vi "Place HDI.vi"(8 "error in (no error)":errorcluster, 9 "Slot Number":dbl, 10 "Chuck Number":dbl, 11 "PickupTool Class in":refnum<class "PickupTool Class.lvclass">) -> (0 "error out":errorcluster, 3 "PickupTool Class out":refnum<class "PickupTool Class.lvclass">)   [LabVIEW 2011, in "PickupTool Class.lvclass"]
uses:
  PickupTool Class.lvclass
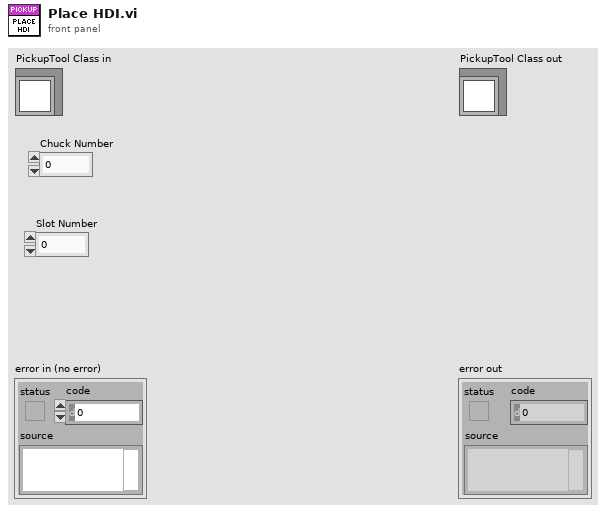
[diagram p1: front panel]
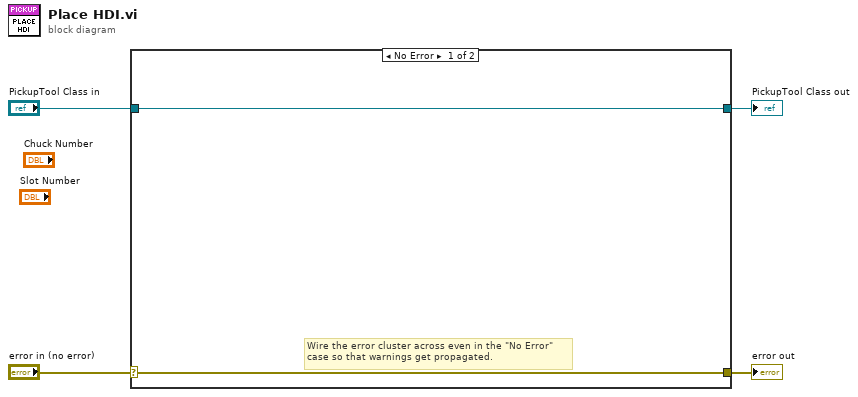
[diagram p0: block diagram]
diagram:
  n1 = case shown="No Error" "error in (no error)" {
    selector: "error in (no error)" -> [w5 w8]
    tunnel: [w5 w8] -> w3
    tunnel: [w6 w7] -> w1
    tunnel: "PickupTool Class in" -> [w6 w7]
    frame No Error {
      # "Wire the error cluster across even in the \"No Error\"\ncase so that warnings get propagated."
    }
    frame Error {
    }
  }
  "error out" <- w3
  "PickupTool Class out" <- w1
